vi "简易PT 100 阻值温度转换器.vi"() -> ()   [LabVIEW 2012]
uses:
  <vilib>/Analysis/1siggen.llb/Ramp Pattern by Samples.vi
  PT 100 Temp Convert to R 1D(dbl).vi
  <vilib>/Analysis/NI_AALBase.lvlib
panel:
  out "数据有效":bool
  in  "选择":enum32{"温度转换为阻值", "阻值转换为温度"}(radio)
  in  "停止":bool
  out "输出值":dbl[](array[numeric])
  in  "输入值":dbl[](array[numeric])
  out "R and Temp":cluster{dbl, dbl}[](graph)
  # "温度范围：-200~850"
  # "℃"
  # "阻值范围：20.5~390"
  # "Ω"
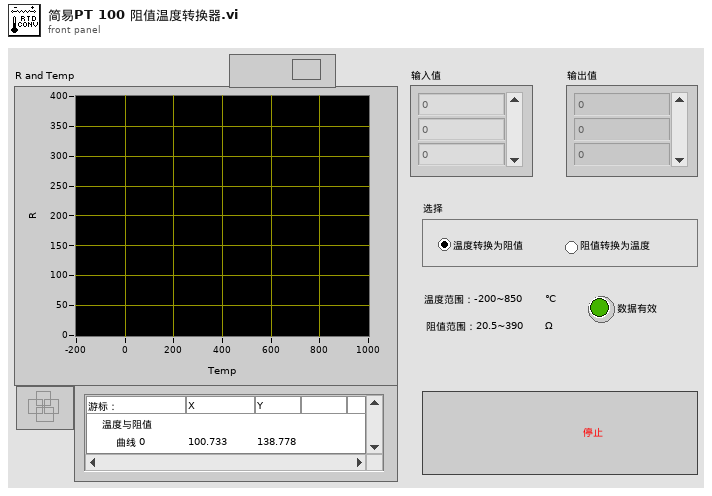
[diagram p1: front panel]
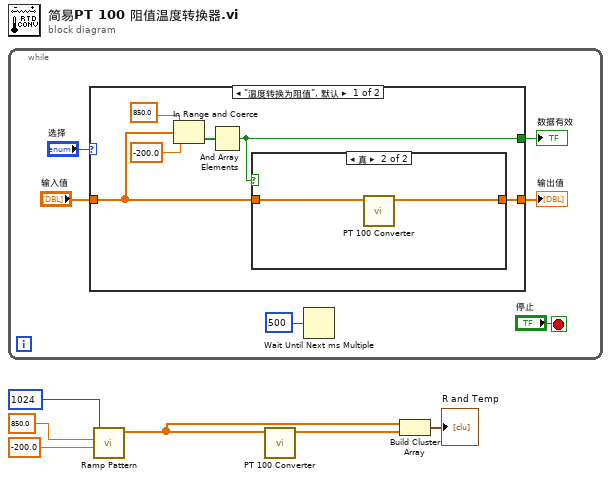
[diagram p0: block diagram]
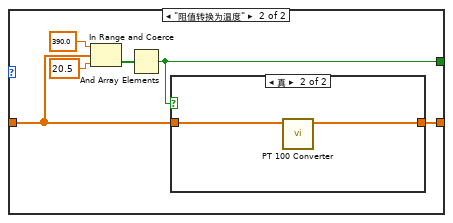
[diagram p3: hidden frame]
diagram:
  n1 = while {
    stop <- "停止" stop-if-true
    n2 = case shown="\"温度转换为阻值\", 默认" "选择" {
      tunnel: "输入值" -> [w15 w23]
      tunnel: [w14 w22] -> w9
      tunnel: [w13 w21] -> w8
      frame "温度转换为阻值", Default {
        n3 = In Range and Coerce(upper limit=850.0, x=w15, lower limit=-200.0) -> (In Range?=w16:bool[])  [unwired: 1 out]
        n4 = And Array Elements(Boolean array=w16) -> (logical AND=w13:bool)
        n5 = case shown="真" w13 {
          tunnel: w15 -> [_ w20]
          tunnel: [_ w19] -> w14
          frame False {
          }
          frame True {
            n6 = call-poly "PT 100 Converter.vi"("t"=w20) -> ("Rt"=w19:dbl[])  [unwired: 10 in]
          }
        }
      }
      frame "阻值转换为温度" {
        n7 = In Range and Coerce(upper limit=390.0 ("上限"), x=w23, lower limit=20.5 ("下限")) -> (In Range?=w24:bool[])  [unwired: 1 out]
        n8 = And Array Elements(Boolean array=w24) -> (logical AND=w21:bool)
        n9 = case shown="真" w21 {
          tunnel: w23 -> [_ w28]
          tunnel: [_ w27] -> w22
          frame False {
          }
          frame True {
            n10 = call-poly "PT 100 Converter.vi"("t"=w28) -> ("Rt"=w27:dbl[])  [unwired: 10 in]
          }
        }
      }
    }
    "输出值" <- w9
    "数据有效" <- w8
    n11 = Wait Until Next ms Multiple(millisecond multiple=u32 500 ("毫秒倍数")) -> ()  [unwired: 1 out]
  }
  n12 = call-poly <vilib>:"Ramp Pattern.vi"("start"=-200.0, "end"=850.0, "samples"=1024) -> ("Ramp Pattern"=w4:dbl[])  [unwired: 7 in, 1 out]
  n13 = call-poly "PT 100 Converter.vi"("t"=w4) -> ("Rt"=w3:dbl[])  [unwired: 10 in]
  n14 = Build Cluster Array(w4, w3) -> (→"R and Temp":cluster{dbl, "Numeric":dbl}[])
